vi "Assemble TabbedViewManager.vi"(9 "View Names":string[](array[string]), 10 "Views":refnum<class "IViewable.lvclass">[](array[class])) -> (3 "TabbedViewManager Out":refnum<class "TabbedViewManager.lvclass">)   [LabVIEW 2017, in "TabbedViewManager.lvlib" / "TabbedViewManager.lvclass"]
doc: "<License>\nCopyright © 2017 Composed Systems, LLC | All rights reserved\nwww.composed.io\n\nAuthor: Ethan Stern <ethan.stern@composed.io>\n\nThis software is provided \"AS IS\" WITHOUT WARRANTIES, either express or implied, AND IS FOR EDUCATIONAL PURPOSES ONLY.\n</License>"
uses:
  TabbedViewManager.lvclass
  C:/Git/mva-framework/Source/Framework/IViewManager/IViewManager/IViewManager.lvclass
  Framework/IViewable/IViewable/IViewable.lvclass
  Framework/IViewable/IViewable/IViewable.lvclass/IViewable.ctl
  Framework/IViewManager/IViewManager Messages/Launch Nested Views Msg/Launch Nested Views Msg.lvclass/Launch Nested Views Msg.ctl
  Framework/IViewManager/IViewManager/IViewManager.lvclass/IViewManager.ctl
  Framework/IViewManager/IViewManager Messages/Launch Nested Views Msg/Pack Launch Nested Views Msg.vi
  <vilib>/Utility/LVClass/Get LV Class Name.vi
  Framework/IViewManager/IViewManager Messages/Launch Nested Views Msg/Launch Nested Views Msg.lvclass
  Framework/IViewManager/IViewManager/IViewManager.lvclass
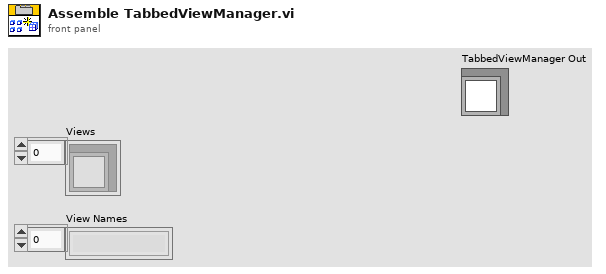
[diagram p1: front panel]
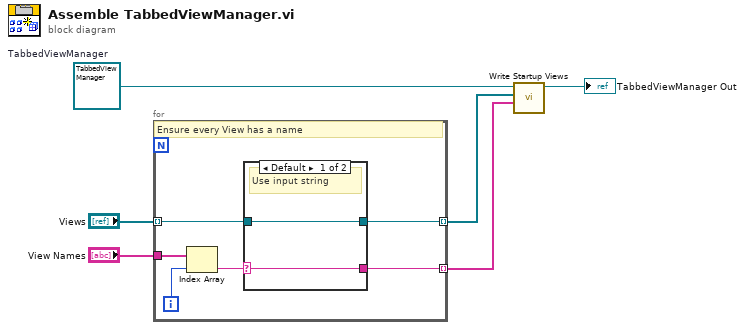
[diagram p0: block diagram]
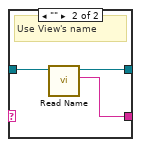
[diagram p2: hidden frame]
diagram:
  w6 = refnum<class "TabbedViewManager.lvclass"> refnum  # TabbedViewManager
  n1 = for {
    tunnel: "Views" -> [w12] mode=indexing
    tunnel: "View Names" -> [w10]
    tunnel: [w11] -> w2 mode=indexing
    tunnel: [w7] -> w1 mode=indexing
    i -> [w8]
    # "Ensure every View has a name"
    n2 = Index Array(array=w10, index=w8) -> (element=w9:string)
    n3 = case shown="Default" w9 {
      selector: w9 -> [w13 _]
      tunnel: w12 -> [w14 w17]
      tunnel: [w14 w16] -> w11
      tunnel: [w13 w15] -> w7
      frame Default {
        # "Use input string"
      }
      frame "" {
        # "Use View's name"
        n4 = call "Read Name.vi"("IViewable In"=w17) -> ("Name"=w15:string, "IViewable Out"=w16:refnum<class "IViewable.lvclass">)  [unwired: 8 in, 1 out]
      }
    }
  }
  n5 = call "Write Startup Views.vi"("View Labels"=w1, "Startup Views"=w2, "IViewManager in"=w6) -> ("IViewManager out"=→"TabbedViewManager Out":refnum<class "TabbedViewManager.lvclass">)  [unwired: 8 in]
